vi "Periodic Tasks.vi"(8 "error in (no error)":errorcluster) -> ()   [LabVIEW 2016]
doc: "This VI runs in parallel to other tasks. It can contain as many user-defined periodic loops as you need. These can carry out PID or other sorts of timed response."
uses:
  <vilib>/Rock Robotics/WPI/DriverStation/WPI_DriverStationRobotMode2.ctl
  <vilib>/Rock Robotics/WPI/Ultrasonic/WPI_UltrasonicRangeUnits.ctl
  <vilib>/Rock Robotics/WPI/ThirdParty/Sensors/navX/_TypeDefs/FRIC_navX_DeviceNumbersTypeDef.ctl
  <vilib>/Rock Robotics/SystemInterfaces/i2clib/i2c_bus.ctl
  <vilib>/Rock Robotics/Network Tables/NT Read Numeric Array.vi
  Robot Global Data.vi
  <vilib>/Rock Robotics/Network Tables/NT Write Number.vi
  <vilib>/Rock Robotics/WPI/Ultrasonic/WPI_SonarSRF04DigitalRefNum Registry Get.vi
  <vilib>/Rock Robotics/WPI/Ultrasonic/WPI_SonarSRF04DigitalGetRange.vi
  US Data.vi
  <vilib>/Rock Robotics/WPI/ThirdParty/Sensors/navX/_Processing Loop/FRIC_navX_Internal_I2C_ProcessingLoop.vi
  <vilib>/Rock Robotics/Network Tables/NT Write Numeric Array.vi
panel:
  out "data out 2":string
  out "x*y 2":dbl
  out "x*y":dbl
  out "Distance Good?":bool
  out "Angle":dbl
  out "Right Distance":dbl
  out "Left Distance":dbl
  out "data out":string
  out "Pose When Pictrue Was Taken":dbl[](array[numeric])
  out "New Pose History":dbl[][](array[numeric])
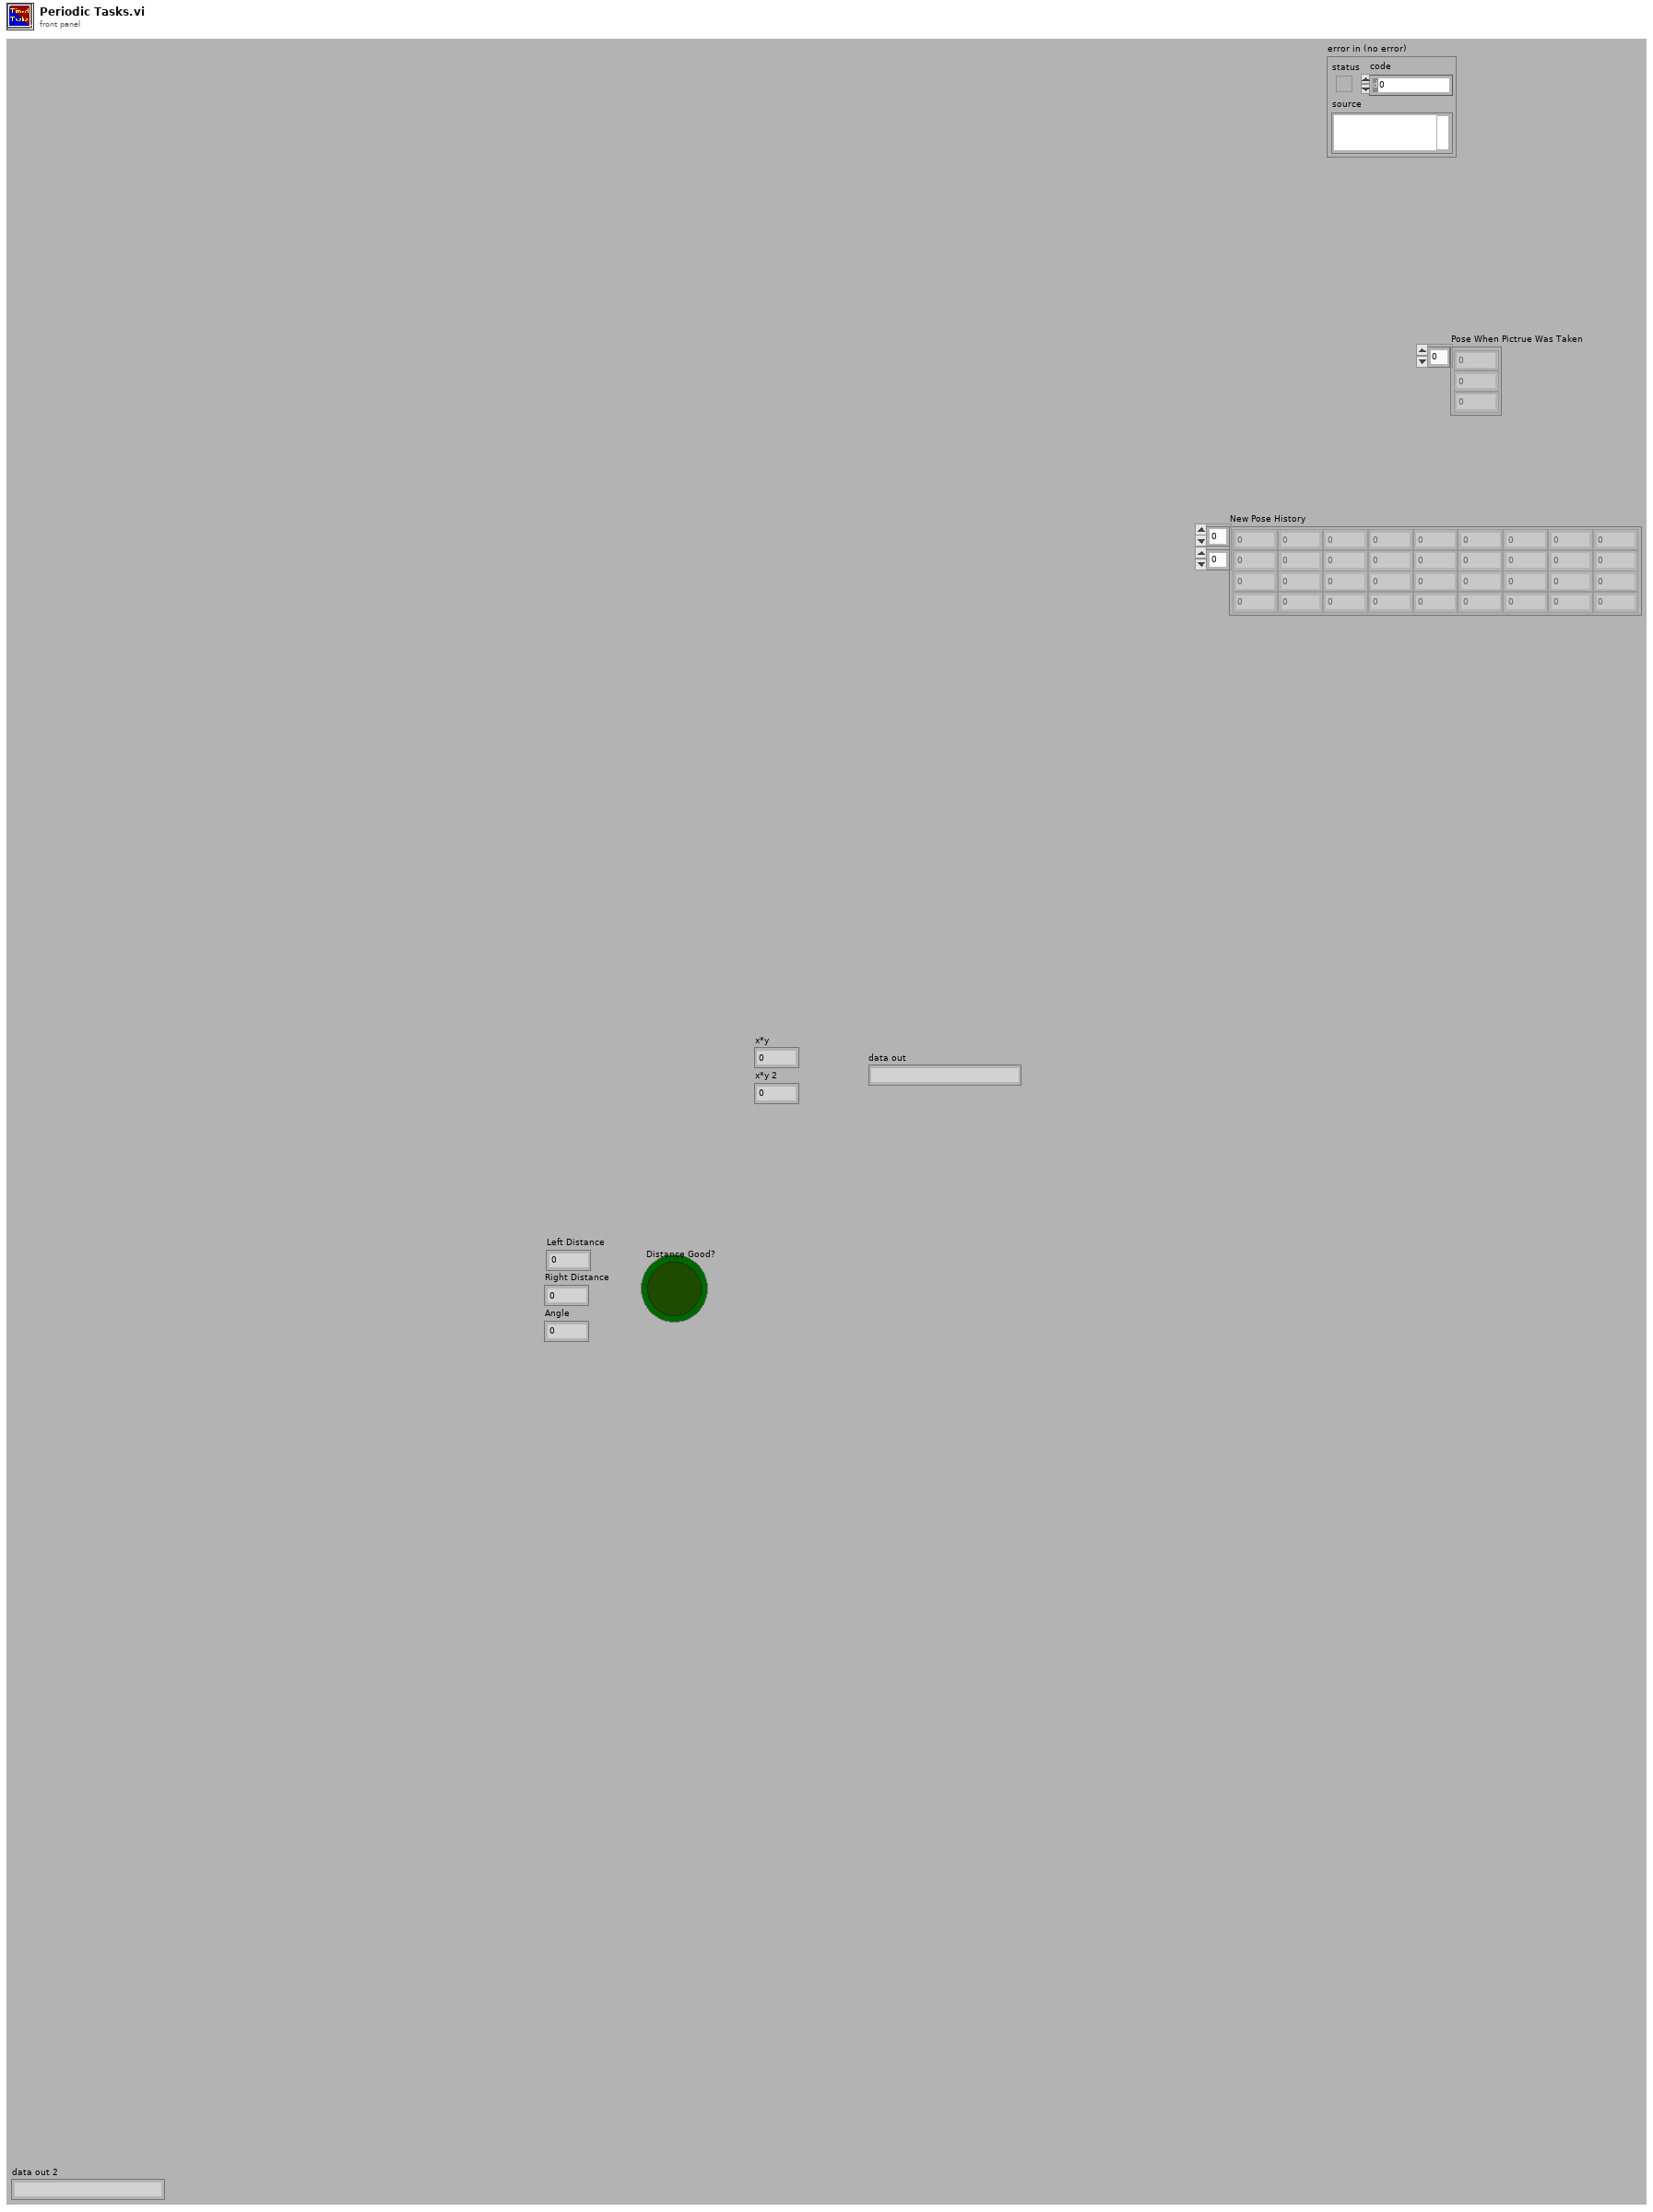
[diagram p1: front panel]
types:
  T1 = typedef "i2c_bus.ctl" = enum16{"I2C On-Board", "I2C MXP", "Invalid"}
  T2 = typedef "FRIC_navX_DeviceNumbersTypeDef.ctl" = enum16{"Dev0", "Dev1", "Dev2", "Dev3"}
  T3 = typedef "WPI_DriverStationRobotMode2.ctl" = enum16{"Autonomous Disabled", "Autonomous Enabled", "Teleop Disabled", "Teleop Enabled", "Disconnected", "Finish", "Test Disabled", "Test Enabled", "Emergency Stopped"}
  T4 = cluster{"Forward Throttle":dbl, "Backward Throttle":dbl, "Rotation Throttle":dbl, "Keep Pose":bool, "Keep Angle":bool, "Slow Drive":bool, "Change Gear Button":bool, "Segway Mode":bool, "Drive to Target":bool, "Y Axis":dbl, "Drive Only Forward":bool}
  T5 = cluster{"Right Button":bool, "Left Button ":bool, "Y":bool, "B":bool, "A":bool, "X":bool, "Left Stick X":dbl, "Left Stick Y":dbl, "Right Stick X ":dbl, "Right Stick Y ":dbl, "Center Left":bool, "Center Right":bool, "Right Stick Touch":bool, "Left Stick Touch ":bool, "Arrows":i16, "Left Throttle":dbl, "Right Throttle":dbl}
  T6 = cluster{"Left Axis":dbl, "Right Axis":dbl, " Encoder Left":dbl, " Encoder Right":dbl, " Navx Fused Heading":dbl, " Navx Pitch":dbl, "Keep Angle":bool, "Keep Pose":bool, "Change Gear Button":bool, "Drive to Target":bool, "Slow Drive":bool, "Segway Mode":bool, "US Right":dbl, "US Left":dbl, "Drive Only Forward":bool}
  T7 = cluster{"Left Axis":dbl, "Right Axis":dbl, "Keep Pose":bool, " Encoder Left":dbl, " Encoder Right":dbl, "High Gear":bool, " Navx Fused Heading":dbl, "Auto Aim":bool, "Angle Difference To Align":dbl, "Keep Angle":bool, "pose X":dbl, "pose Y":dbl, "Drive to Target":bool, "Slow Drive":bool, "Segway Mode":bool, " Navx Pitch":dbl, "US Right":dbl, "US Left":dbl, "Drive Only Forward":bool}
  T8 = typedef "WPI_UltrasonicRangeUnits.ctl" = enum16{"inches", "mm"}
  T9 = typedef "WPI_UltrasonicDeviceRef.ctl" = cluster{"DevStatus":errorcluster, "Ping Channel":T10, "Echo Channel":T10, "CntIndex":T11}
  T10 = typedef "FPGA_DIOChannel.ctl" = enum8{"DIO 0", "DIO 1", "DIO 2", "DIO 3", "DIO 4", "DIO 5", "DIO 6", "DIO 7", "DIO 8", "DIO 9", "DIO MXP 0", "DIO MXP 1", "DIO MXP 2", "DIO MXP 3", "DIO MXP 4", "DIO MXP 5", "DIO MXP 6", "DIO MXP 7", "DIO MXP 8", "DIO MXP 9", "DIO MXP 10", "DIO MXP 11", "DIO MXP 12", "DIO MXP 13", "DIO MXP 14", "DIO MXP 15", "SPI Port CS1", "SPI Port CS2", "SPI Port CS3", "SPI Port MISO", "SPI Port MOSI", "Invalid"}
  T11 = typedef "FPGA_CounterCtrSystemIndex.ctl" = enum8{"Ctr 0", "Ctr 1", "Ctr 2", "Ctr 3", "Ctr 4", "Ctr 5", "Ctr 6", "Ctr 7", "Invalid"}
  T12 = cluster{"Yaw":dbl, "Roll":dbl, "Pitch":dbl, "Heading":dbl, "Fused Heading":dbl}
  T13 = typedef "WPI_EncoderDevRef.ctl" = cluster{"DevStatus":errorcluster, "EncoderIndex":T14, "CounterIndex":T11, "DistancePerCount":dbl, "Decoding Type":T15}
  T14 = typedef "FPGA_EncoderIdx.ctl" = enum8{"Enc 0", "Enc 1", "Enc 2", "Enc 3", "Enc 4", "Enc 5", "Enc 6", "Enc 7", "Invalid"}
  T15 = typedef "WPI_EncoderType.ctl" = enum16{"1x", "2x", "4x"}
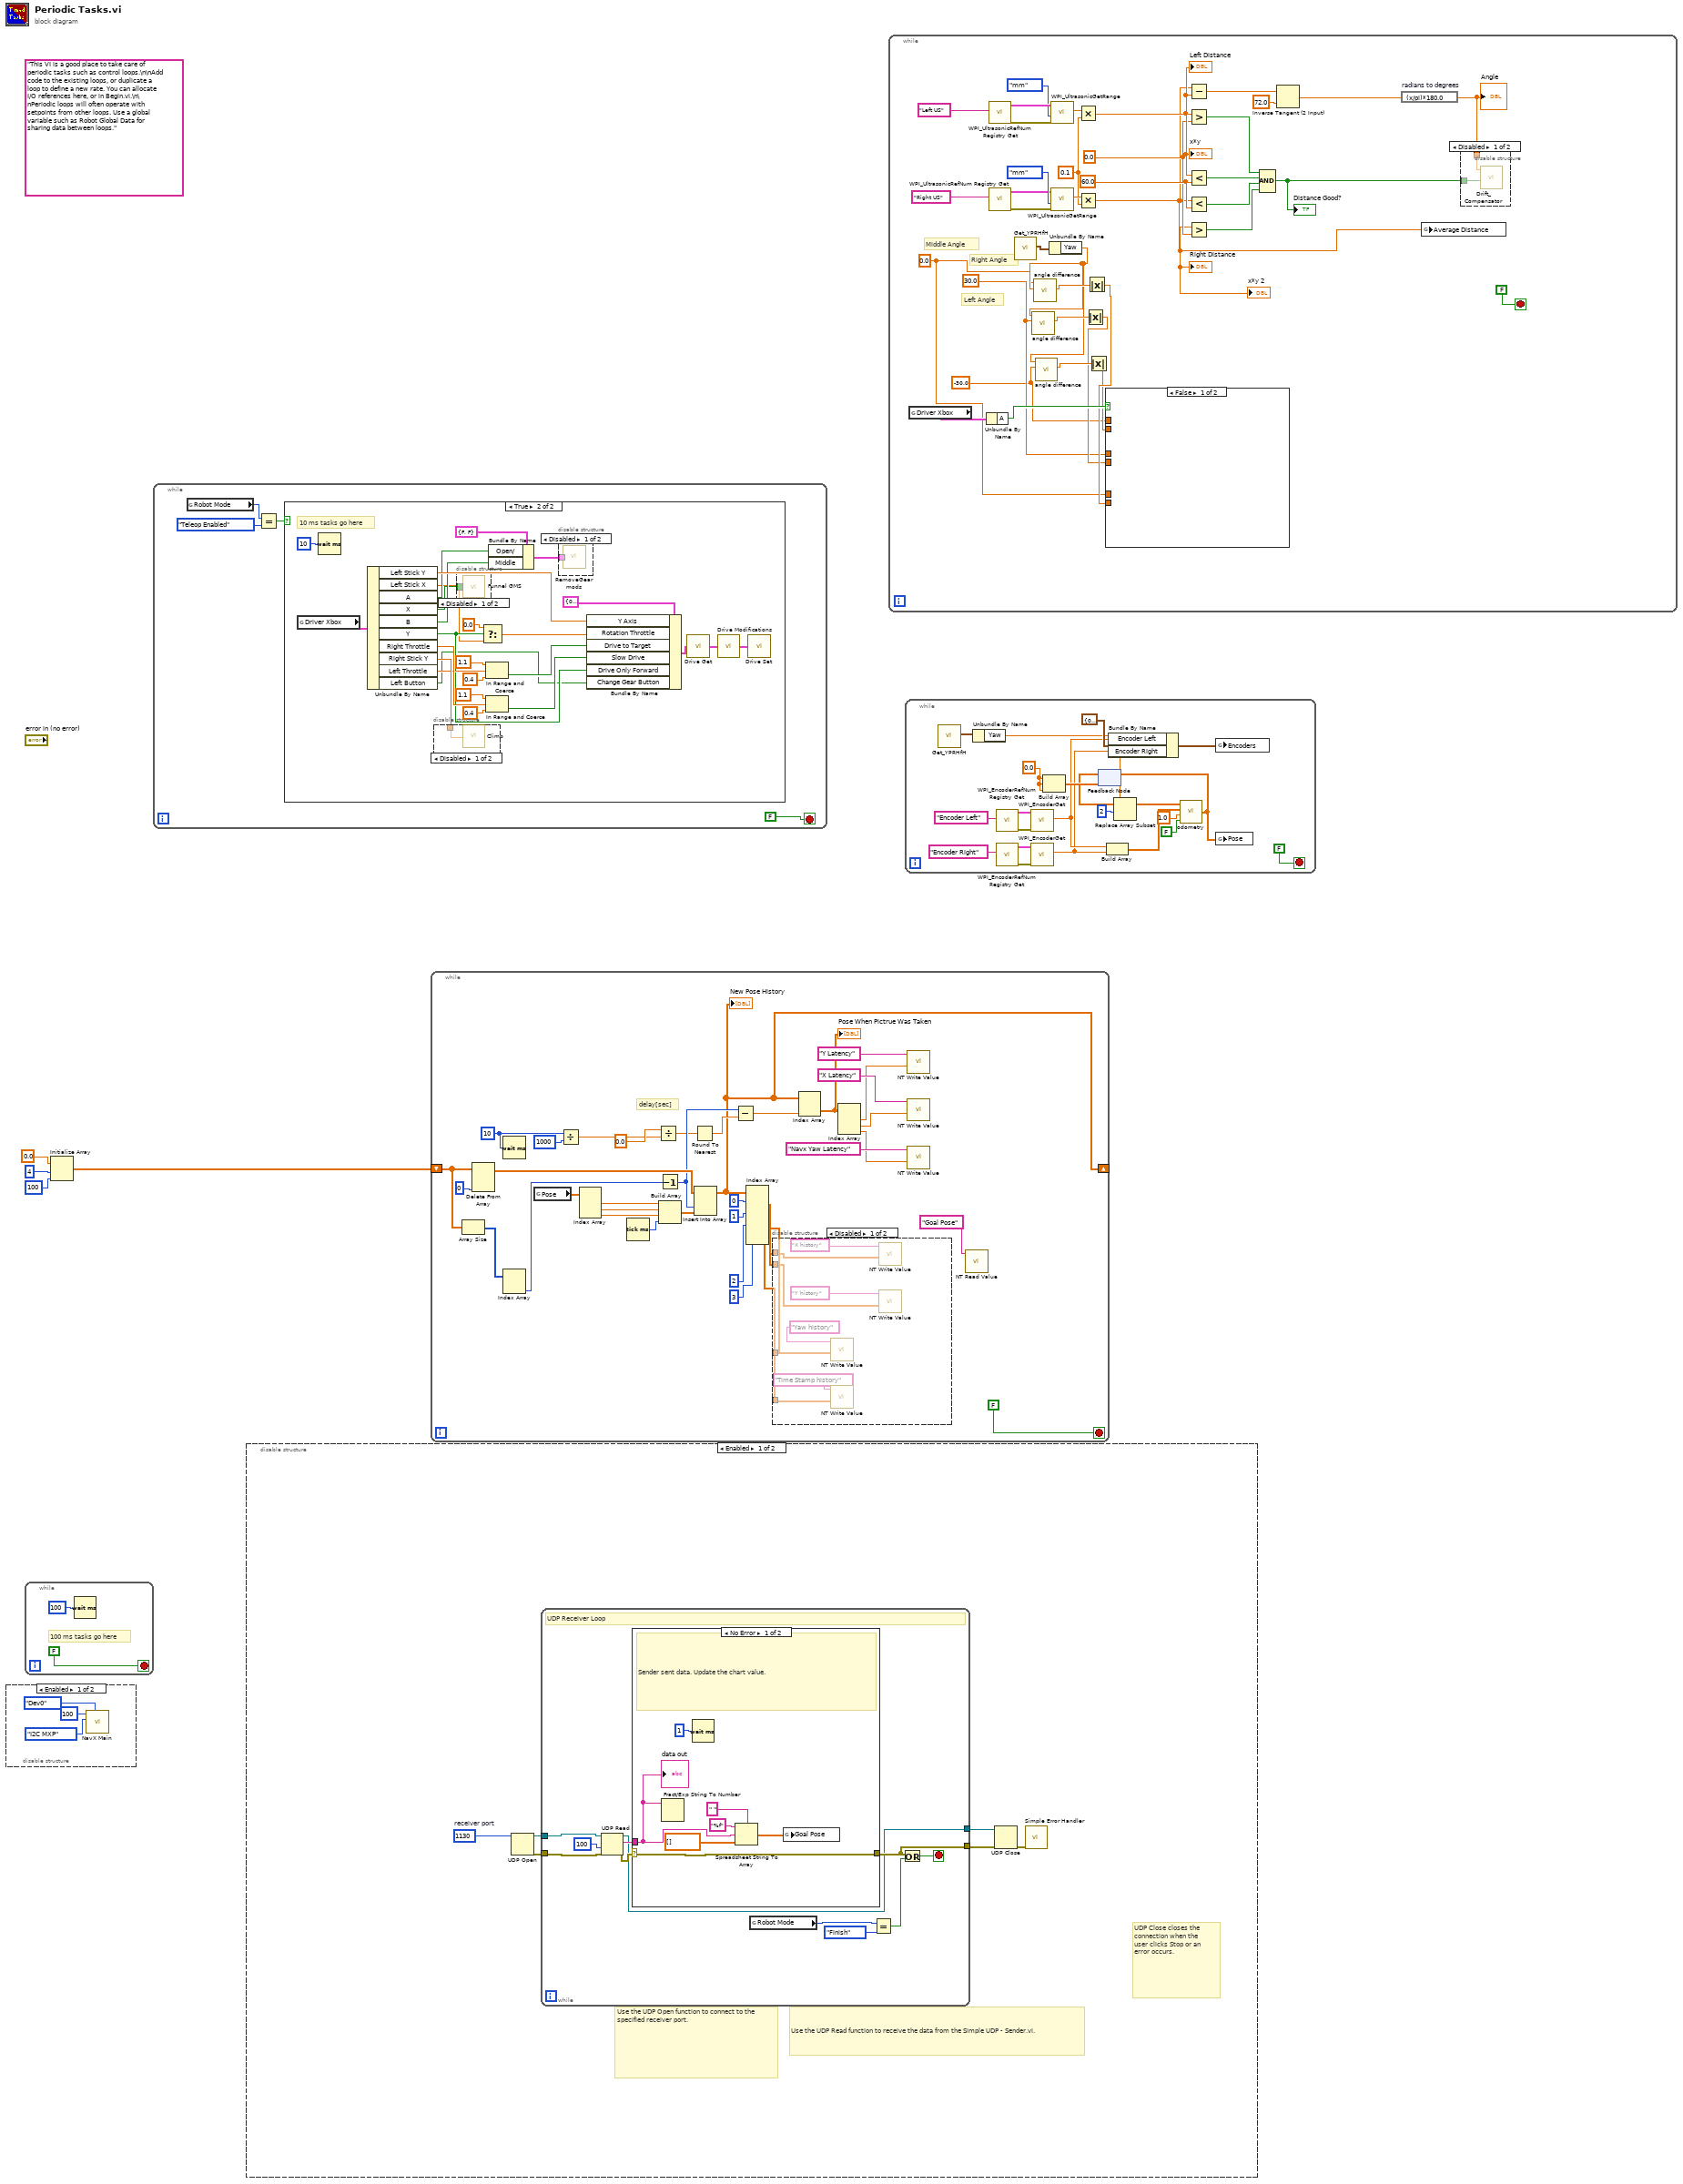
[diagram p0: block diagram]
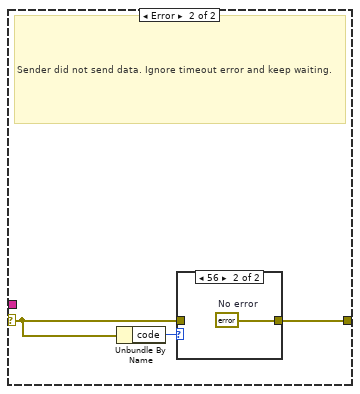
[diagram p3: hidden frame]
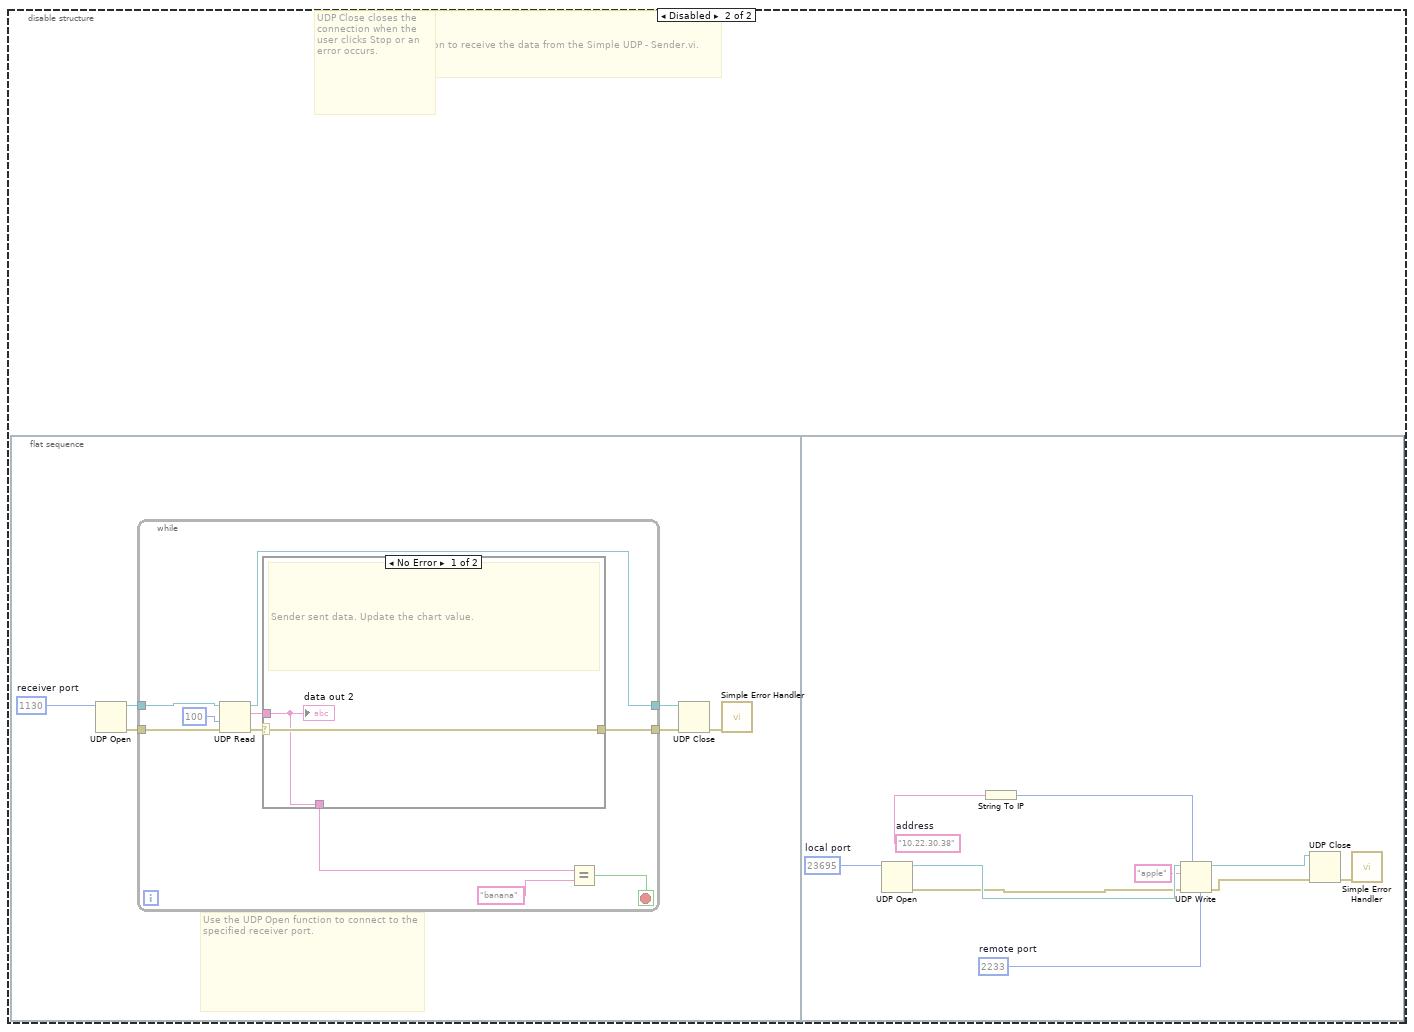
[diagram p5: hidden frame]
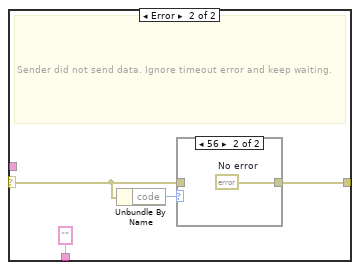
[diagram p6: hidden frame]
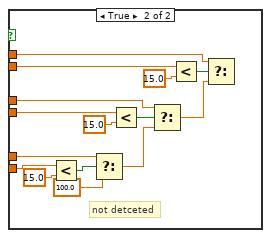
[diagram p8: hidden frame]
diagram:
  (unwired) "This VI is a good place to take care of periodic tasks such as control loops.\n\nAdd code to the existing loops, or duplicate a loop to define a new rate. You can allocate I/O references here, or in Begin.vi.\n\nPeriodic loops will often operate with setpoints from other loops. Use a global variable such as Robot Global Data for sharing data between loops."
  n1 = disable-structure shown="Enabled" {
    frame Enabled {
      n2 = call-poly <vilib>:"NavX Main.vi"("Device Number"=FRIC_navX_DeviceNumbersTypeDef."Dev0", "I2C Bus"=i2c_bus."I2C MXP", "Rate (4Hz-200Hz)"=u8 100) -> ()  [unwired: 9 in]
    }
    frame Disabled {
    }
  }
  n3 = while {
    stop <- FALSE stop-if-true
    # "100 ms tasks go here"
    n4 = Wait (ms)(milliseconds to wait=u32 100) -> ()  [unwired: 1 out]
  }
  n5 = Initialize Array(0.0 ("element"), 4 ("dimension size"), 100 ("dimension size")) -> (w1:dbl[][])
  n6 = while {
    stop <- FALSE stop-if-true
    n7 = global read "Robot Global Data.vi" "Robot Mode"() -> (w12:T3)
    n8 = Equal?(x=w12, y=WPI_DriverStationRobotMode2."Teleop Enabled") -> (x = y?=w10:bool)
    n9 = case shown="True" w10 {
      frame False {
      }
      frame True {
        # "10 ms tasks go here"
        n10 = global read "Robot Global Data.vi" "Driver Xbox"() -> (w36:T5)
        n11 = Wait (ms)(milliseconds to wait=u32 10) -> ()  [unwired: 1 out]
        n12 = Unbundle By Name(w36) -> ("Left Stick Y"=w37:dbl, "Left Stick X"=w16:dbl, "A"=w33:bool, "X"=w30:bool, "B"=w32:bool, "Y"=w18:bool, "Right Throttle"=w22:dbl, "Right Stick Y"=w31:dbl, "Left Throttle"=w21:dbl, "Left Button"=w14:bool)
        n13 = disable-structure shown="Disabled" {
          disable-tunnel: w31 -> [w40 _]
          frame Disabled {
            n14 = call "Climb.vi"("Climb motor value"=w40) -> ()  [unwired: 1 in]
          }
          frame Enabled {
          }
        }
        n15 = disable-structure shown="Disabled" {
          disable-tunnel: w30 -> [w41 _]
          frame Disabled {
            n16 = call "Funnel GMS.vi"("Open Solenoid"=w41) -> ()  [unwired: 1 in]
          }
          frame Enabled {
          }
        }
        n17 = Select(t=0.0, s=w18, f=w16) -> (s? t:f=w15:dbl)
        n18 = In Range and Coerce(upper limit=1.1, x=w21, lower limit=0.4) -> (In Range?=w20:bool)  [unwired: 1 out]
        n19 = In Range and Coerce(upper limit=1.1, x=w22, lower limit=0.4) -> (In Range?=w25:bool)  [unwired: 1 out]
        n20 = Bundle By Name(cluster=cluster{"Open/":bool, "Middle ":bool} {"Open/"=FALSE, "Middle "=FALSE} ("xbox data"), "Open/"=w33, "Middle"=w32) -> (w34:cluster{"Open/":bool, "Middle ":bool})
        n21 = disable-structure shown="Disabled" {
          disable-tunnel: w34 -> [w42 _]
          frame Disabled {
            n22 = call "RemoveGear mods.vi"("xbox data"=w42) -> ()  [unwired: 1 in]
          }
          frame Enabled {
          }
        }
        n23 = Bundle By Name(cluster=T4 {"Forward Throttle"=0.0, "Backward Throttle"=0.0, "Rotation Throttle"=0.0, "Keep Pose"=FALSE, "Keep Angle"=FALSE, "Slow Drive"=FALSE, "Change Gear Button"=FALSE, "Segway Mode"=FALSE, "Drive to Target"=FALSE, "Y Axis"=0.0, "Drive Only Forward"=FALSE} ("Joystick In"), "Y Axis"=w37, "Rotation Throttle"=w15, "Drive to Target"=w20, "Slow Drive"=w25, "Drive Only Forward"=w18, "Change Gear Button"=w14) -> (w28:T4)
        n24 = call "Drive Get.vi"("Joystick In"=w28) -> ("Get Out"=w38:T6)
        n25 = call "Drive Modifications.vi"("Mods In"=w38) -> ("Mods Out"=w19:T7)
        n26 = call "Drive Set.vi"("Set In"=w19) -> ()  [unwired: 1 in]
      }
    }
  }
  n27 = disable-structure shown="Enabled" {
    frame Enabled {
      w43 = u16 1130  # receiver port
      # "UDP Close closes the connection when the user clicks Stop or an error occurs."
      # "Use the UDP Open function to connect to the specified receiver port."
      # "Use the UDP Read function to receive the data from the Simple UDP - Sender.vi."
      n28 = UDP Open(11:w43) -> (port=w44:refnum<k16>, 0:w45:errorcluster)  [unwired: 4 in, 1 out]
      n29 = while {
        tunnel: w44 -> [w59]
        tunnel: [w52] -> w48
        tunnel: w45 -> [w57]
        tunnel: [w53] -> w46
        stop <- w58 stop-if-true
        # "UDP Receiver Loop"
        n30 = UDP Read(connection ID=w59, timeout ms (25000)=100, 8:w57) -> (data out=w55:string, error out=w54:errorcluster, 3:w52:refnum<k16>)  [unwired: 3 out]
        n31 = case shown="No Error" w54 {
          selector: w54 -> [w66 w68]
          tunnel: w55 -> [w65 _]
          tunnel: [w66 w67] -> w53
          frame No Error {
            # "Sender sent data. Update the chart value."
            n32 = Fract/Exp String To Number(string=w65) -> ()  [unwired: 3 in, 2 out]
            n33 = Wait (ms)(milliseconds to wait=u32 1) -> ()  [unwired: 1 out]
            n34 = Spreadsheet String To Array(delimiter (Tab)=" ", format string="%f", spreadsheet string=w65, array type (2D Dbl)=dbl[] []) -> (array=w61:dbl[])
            n35 = global write "Robot Global Data.vi" "Goal Pose"(w61) -> ()
            "data out" <- w65
          }
          frame Error {
            # "Sender did not send data. Ignore timeout error and keep waiting."
            n36 = Unbundle By Name(w68) -> ("code"=w69:i32)
            n37 = case shown="56" w69 {
              tunnel: w68 -> [w70 _]
              tunnel: [w70 w71] -> w67
              frame Default {
              }
              frame 56 {
                w71 = errorcluster {"status"=FALSE, "code"=0, "source"=""}  # No error
              }
            }
          }
        }
        n38 = global read "Robot Global Data.vi" "Robot Mode"() -> (w51:T3)
        n39 = Equal?(x=w51, y=WPI_DriverStationRobotMode2."Finish" ("Robot Mode")) -> (x = y?=w49:bool)
        n40 = Or(x=w53, y=w49) -> (x .or. y?=w58:bool)
      }
      n41 = UDP Close(connection ID=w48, 8:w46) -> (error out=w47:errorcluster)  [unwired: 1 out]
      n42 = call <vilib>:"Simple Error Handler.vi"("error in (no error)"=w47) -> ()  [unwired: 1 in, 8 out]
    }
    frame Disabled {
      # "UDP Close closes the connection when the user clicks Stop or an error occurs."
      # "Use the UDP Read function to receive the data from the Simple UDP - Sender.vi."
      n43 = flat-sequence {
        frame #0 {
          w72 = u16 1130  # receiver port
          # "Use the UDP Open function to connect to the specified receiver port."
          n44 = UDP Open(11:w72) -> (port=w73:refnum<k16>, 0:w74:errorcluster)  [unwired: 4 in, 1 out]
          n45 = while {
            tunnel: w74 -> [w85]
            tunnel: [w86] -> w75
            tunnel: w73 -> [w84]
            tunnel: [w87] -> w77
            stop <- w80 stop-if-true
            n46 = UDP Read(connection ID=w84, timeout ms (25000)=100, 8:w85) -> (data out=w82:string, error out=w81:errorcluster, 3:w87:refnum<k16>)  [unwired: 3 out]
            n47 = case shown="No Error" w81 {
              selector: w81 -> [w89 w92]
              tunnel: w82 -> [w88 _]
              tunnel: [w89 w91] -> w86
              tunnel: [w88 "" ("data out")] -> w78
              frame No Error {
                # "Sender sent data. Update the chart value."
                "data out 2" <- w88
              }
              frame Error {
                # "Sender did not send data. Ignore timeout error and keep waiting."
                n48 = Unbundle By Name(w92) -> ("code"=w93:i32)
                n49 = case shown="56" w93 {
                  tunnel: w92 -> [w94 _]
                  tunnel: [w94 w95] -> w91
                  frame Default {
                  }
                  frame 56 {
                    w95 = errorcluster {"status"=FALSE, "code"=0, "source"=""}  # No error
                  }
                }
              }
            }
            n50 = Equal?(x=w78, y="banana" ("data out 3")) -> (x = y?=w80:bool)
          }
          n51 = UDP Close(connection ID=w77, 8:w75) -> (error out=w76:errorcluster)  [unwired: 1 out]
          n52 = call <vilib>:"Simple Error Handler.vi"("error in (no error)"=w76) -> ()  [unwired: 1 in, 8 out]
        }
        frame #1 {
          w97 = u16 2233  # remote port
          w98 = u16 23695  # local port
          w103 = "10.22.30.38"  # address
          n53 = UDP Open(11:w98) -> (port=w100:refnum<k16>, 0:w99:errorcluster)  [unwired: 4 in, 1 out]
          n54 = String To IP(1:w103) -> (0:w101:u32)
          n55 = UDP Write(address=w101, port or service name=w97, connection ID=w100, data in="apple", 8:w99) -> (error out=w104:errorcluster, 3:w105:refnum<k16>)  [unwired: 1 in]
          n56 = UDP Close(connection ID=w105, 8:w104) -> (error out=w102:errorcluster)  [unwired: 1 out]
          n57 = call <vilib>:"Simple Error Handler.vi"("error in (no error)"=w102) -> ()  [unwired: 4 in, 5 out]
        }
      }
    }
  }
  n58 = while {
    shift-right: [w115] -> _
    shift-left: w1 -> [w137]
    stop <- FALSE stop-if-true
    w136 = u32 10 ("milliseconds to wait")
    # "delay[sec]"
    n59 = Array Size(array=w137) -> (size(s)=w142:i32[])
    n60 = Delete From Array(array=w137, index (col)=0 ("disabled index (col)")) -> (array with subset deleted=w140:dbl[][])  [unwired: 2 in, 1 out]
    n61 = Wait (ms)(milliseconds to wait=w136) -> ()  [unwired: 1 out]
    n62 = Index Array(array=w142) -> (element #2=w141:i32)  [unwired: 2 in, 1 out]
    n63 = global read "Robot Global Data.vi" "Pose"() -> (w121:dbl[])
    n64 = Divide(x=w136, y=u32 1000) -> (x/y=w133:dbl)
    n65 = Index Array(array=w121) -> (element #1=w120:dbl, element #2=w119:dbl, element #3=w118:dbl)  [unwired: 3 in]
    n66 = Tick Count (ms)() -> (millisecond timer value=w117:u32)
    n67 = Divide(x=0.0 ("Delay[sec]"), y=w133) -> (x/y=w131:dbl)
    n68 = Decrement(x=w141) -> (x-1=w132:i32)
    n69 = Build Array(w120, w119, w118, w117) -> (w116:dbl[])
    n70 = Round To Nearest(number=w131) -> (nearest integer value=w130:dbl)
    n71 = Insert Into Array(array=w140, index (col)=w132, new element=w116) -> (w115:dbl[][])  [unwired: 1 in]
    "New Pose History" <- w115
    n72 = Subtract(x=w132, y=w130) -> (x-y=w129:dbl)
    n73 = Index Array(array=w115, index (row) #1=0 ("index (row)"), index (row) #2=1 ("index (row)"), index (row) #3=2 ("index (row)"), index (row) #4=3 ("index (row)")) -> (element #1=w113:dbl[], element #2=w109:dbl[], element #3=w108:dbl[], element #4=w107:dbl[])  [unwired: 4 in]
    n74 = disable-structure shown="Disabled" {
      disable-tunnel: w113 -> [w150 _]
      disable-tunnel: w109 -> [w145 _]
      disable-tunnel: w108 -> [w144 _]
      disable-tunnel: w107 -> [w143 _]
      frame Disabled {
        n75 = call-poly <vilib>:"NT Write Value.vi"("Numeric Array"=w144, "Name"="Yaw history") -> ()  [unwired: 9 in, 1 out]
        n76 = call-poly <vilib>:"NT Write Value.vi"("Numeric Array"=w143, "Name"="Time Stamp history") -> ()  [unwired: 9 in, 1 out]
        n77 = call-poly <vilib>:"NT Write Value.vi"("Numeric Array"=w150, "Name"="X history") -> ()  [unwired: 9 in, 1 out]
        n78 = call-poly <vilib>:"NT Write Value.vi"("Numeric Array"=w145, "Name"="Y history") -> ()  [unwired: 9 in, 1 out]
      }
      frame Enabled {
      }
    }
    n79 = Index Array(array=w115, index (col)=w129) -> (element=w127:dbl[])  [unwired: 1 in]
    "Pose When Pictrue Was Taken" <- w127
    n80 = Index Array(array=w127) -> (element #1=w123:dbl, element #2=w122:dbl, element #3=w126:dbl)  [unwired: 3 in]
    n81 = call-poly <vilib>:"NT Write Value.vi"("Numeric"=w123, "Name"="Y Latency") -> ()  [unwired: 9 in, 1 out]
    n82 = call-poly <vilib>:"NT Write Value.vi"("Numeric"=w122, "Name"="X Latency") -> ()  [unwired: 9 in, 1 out]
    n83 = call-poly <vilib>:"NT Write Value.vi"("Numeric"=w126, "Name"="Navx Yaw Latency") -> ()  [unwired: 9 in, 1 out]
    n84 = call-poly <vilib>:"NT Read Value.vi"("Name"="Goal Pose") -> ()  [unwired: 9 in, 2 out]
  }
  n85 = while {
    stop <- FALSE stop-if-true
    w151 = -30.0 ("y")
    w153 = 30.0 ("y")
    w155 = 0.0 ("y")
    w186 = 0.1 ("y")
    w179 = 0.0 ("y")
    w180 = 60.0 ("y")
    # "Left Angle"
    # "Right Angle"
    # "Middle Angle"
    n86 = global read "Robot Global Data.vi" "Driver Xbox"() -> (w163:T5)
    n87 = Unbundle By Name(w163) -> ("A"=w162:bool)
    n88 = call-poly <vilib>:"WPI_UltrasonicRefNum Registry Get.vi"("refnum name"="Left US") -> ("error out"=w170:errorcluster, "SonarSRF04DevRef"=w169:T9)  [unwired: 9 in]
    n89 = call-poly <vilib>:"WPI_UltrasonicRefNum Registry Get.vi"("refnum name"="Right US") -> ("error out"=w165:errorcluster, "SonarSRF04DevRef"=w166:T9)  [unwired: 9 in]
    n90 = call <vilib>:"Get_YPRHfH.vi"() -> ("YRPHfH"=w161:T12)  [unwired: 11 in]
    n91 = Unbundle By Name(w161) -> ("Yaw"=w157:dbl)
    n92 = call "angle difference.vi"("angle2"=w153, "angle1"=w157) -> ("angle diff"=w159:dbl)  [unwired: 9 in]
    n93 = call "angle difference.vi"("angle2"=w157, "angle1"=w155) -> ("angle diff"=w160:dbl)  [unwired: 9 in]
    n94 = call "angle difference.vi"("angle2"=w151, "angle1"=w157) -> ("angle diff"=w158:dbl)  [unwired: 9 in]
    n95 = call-poly <vilib>:"WPI_UltrasonicGetRange.vi"("error in (no error)"=w170, "Range Units"=WPI_UltrasonicRangeUnits."mm", "SonarSRF04DevRef"=w169) -> ("Distance"=w188:dbl)  [unwired: 6 in, 2 out]
    n96 = call-poly <vilib>:"WPI_UltrasonicGetRange.vi"("error in (no error)"=w165, "Range Units"=WPI_UltrasonicRangeUnits."mm", "SonarSRF04DevRef"=w166) -> ("Distance"=w187:dbl)  [unwired: 6 in, 2 out]
    n97 = Multiply(x=w188, y=w186) -> (x*y=w181:dbl)
    "Left Distance" <- w181
    "x*y" <- w181
    n98 = Multiply(x=w187, y=w186) -> (x*y=w172:dbl)
    "Right Distance" <- w172
    "x*y 2" <- w172
    n99 = Absolute Value(x=w159) -> (abs(x)=w154:dbl)
    n100 = Absolute Value(x=w160) -> (abs(x)=w156:dbl)
    n101 = Absolute Value(x=w158) -> (abs(x)=w152:dbl)
    n102 = case shown="False" w162 {
      tunnel: w156 -> [_ w194]
      tunnel: w155 -> [_ w201]
      tunnel: w154 -> [_ w199]
      tunnel: w153 -> [_ w197]
      tunnel: w152 -> [_ w192]
      tunnel: w151 -> [_ w190]
      frame False {
      }
      frame True {
        # "not detceted"
        n103 = Less?(x=w194, y=15.0) -> (x < y?=w202:bool)
        n104 = Select(t=w201, s=w202, f=100.0) -> (s? t:f=w196:dbl)
        n105 = Less?(x=w199, y=15.0) -> (x < y?=w198:bool)
        n106 = Select(t=w197, s=w198, f=w196) -> (s? t:f=w191:dbl)
        n107 = Less?(x=w192, y=15.0) -> (x < y?=w195:bool)
        n108 = Select(t=w190, s=w195, f=w191) -> ()  [unwired: 1 out]
      }
    }
    n109 = Subtract(x=w172, y=w181) -> (x-y=w185:dbl)
    n110 = Greater?(x=w181, y=w179) -> (0:w178:bool)
    n111 = Less?(x=w181, y=w180) -> (x < y?=w177:bool)
    n112 = Less?(x=w172, y=w180) -> (x < y?=w176:bool)
    n113 = Greater?(x=w172, y=w179) -> (0:w175:bool)
    n114 = Compound Arithmetic op=AND(w178, w177, w176, w175) -> (w174:bool)
    "Distance Good?" <- w174
    n115 = Inverse Tangent (2 Input)(1:72.0 ("x"), 2:w185) -> (0:w183:dbl)
    n116 = expression code="(x/pi)*180.0" "radians to degrees"(w183) -> (w173:dbl)
    "Angle" <- w173
    n117 = global write "US Data.vi" "Average Distance"(w172) -> ()
    n118 = disable-structure shown="Disabled" {
      disable-tunnel: w174 -> [w205 _]
      disable-tunnel: w173 -> [w204 _]
      frame Disabled {
        n119 = call <vilib>:"Drift_Compensator.vi"("Zero Yaw"=w205, "Raw Yaw"=w204) -> ()  [unwired: 9 in, 1 out]
      }
      frame Enabled {
      }
    }
  }
  n120 = while {
    stop <- FALSE stop-if-true
    w225 = 0.0 ("element")
    n121 = call <vilib>:"Get_YPRHfH.vi"() -> ("YRPHfH"=w207:T12)  [unwired: 11 in]
    n122 = Unbundle By Name(w207) -> ("Yaw"=w206:dbl)
    n123 = call <vilib>:"WPI_EncoderRefNum Registry Get.vi"("refnum name"="Encoder Left") -> ("error out"=w217:errorcluster, "EncoderDevRef"=w216:T13)  [unwired: 9 in]
    n124 = call <vilib>:"WPI_EncoderRefNum Registry Get.vi"("refnum name"="Encoder Right") -> ("error out"=w212:errorcluster, "EncoderDevRef"=w213:T13)  [unwired: 9 in]
    n125 = call <vilib>:"WPI_EncoderGet.vi"("error in (no error)"=w217, "EncoderDevRef"=w216) -> ("Distance"=w209:dbl)  [unwired: 4 in, 5 out]
    n126 = call <vilib>:"WPI_EncoderGet.vi"("error in (no error)"=w212, "EncoderDevRef"=w213) -> ("Distance"=w208:dbl)  [unwired: 4 in, 5 out]
    n127 = Build Array(w225, w225, w225) -> (w226:dbl[])
    n128 = feedback #1(w226) -> (w224:dbl[])
    n129 = Build Array(w209, w208) -> (w218:dbl[])
    n130 = Bundle By Name(cluster=cluster{"Encoder Left":dbl, "Encoder Right":dbl} {"Encoder Left"=0.0, "Encoder Right"=0.0} ("Encoders"), "Encoder Left"=w209, "Encoder Right"=w208) -> (w210:cluster{"Encoder Left":dbl, "Encoder Right":dbl})
    n131 = Replace Array Subset(array=w224, new element=w206, index=2) -> (w221:dbl[])
    n132 = call "odometry.vi"("reset"=FALSE, "distance between sides of wheels"=1.0, "encoders in"=w218, "state in"=w221) -> ("state out"=w219:dbl[])
    n133 = feedback-in #1(w219) -> ()
    n134 = global write "Robot Global Data.vi" "Encoders"(w210) -> ()
    n135 = global write "Robot Global Data.vi" "Pose"(w219) -> ()
  }
